vi "Revealed Content.vi"(8 "error in (no error)":errorcluster, 11 "Bag in":refnum<class "Bag.lvclass">) -> (0 "error out":errorcluster, 2 "Cubes":T1, 3 "Bag out":refnum<class "Bag.lvclass">)   [LabVIEW 2020, in "Bag.lvclass"]
uses:
  Bag.lvclass
  Cubes.ctl
  Bag.lvclass/Bag.ctl
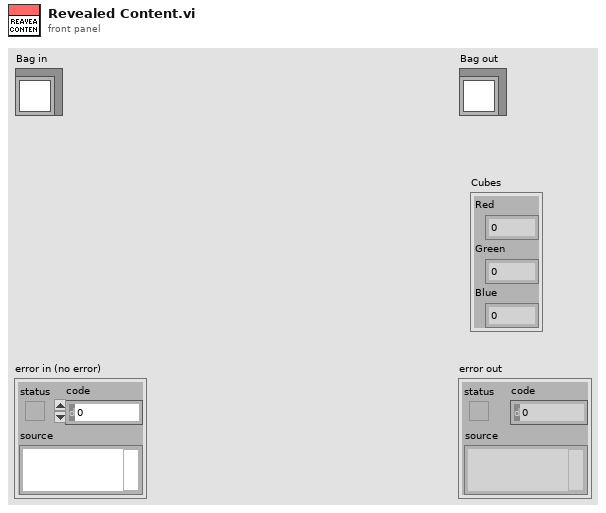
[diagram p1: front panel]
types:
  T1 = typedef "Bag.lvclass/Cubes.ctl" = cluster{"Red":i32, "Green":i32, "Blue":i32}
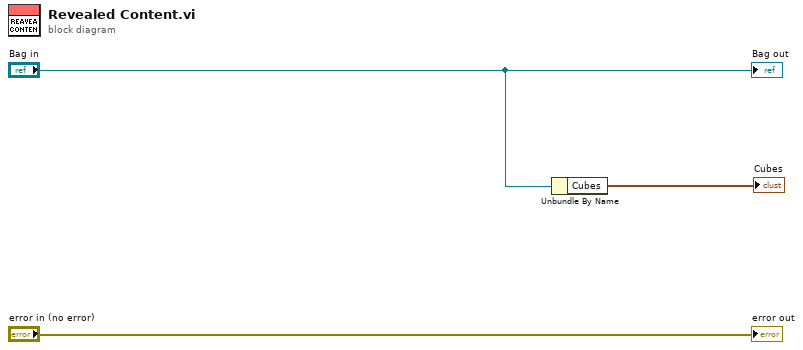
[diagram p0: block diagram]
diagram:
  n1 = Unbundle By Name("Bag in") -> ("Cubes"=→"Cubes":T1)
  "error out" <- "error in (no error)"
  "Bag out" <- "Bag in"
